vi "Share boolean signal.vi"() -> ()   [LabVIEW 2012]
uses:
  <vilib>/Platform/TimedLoop/XDataNode/timing_clust.ctl
  <vilib>/Platform/TimedLoop/XDataNode/nitl_modes.ctl
  <vilib>/Platform/TimedLoop/XDataNode/wakeup.ctl
  <vilib>/rvi/Emulation/niFpgaSctlEmulationRegisterWithScheduler.vi
  <vilib>/rvi/Emulation/niFpgaSctlEmulationScheduler.vi
  <vilib>/Platform/TimedLoop/XDataNode/XDataNode.xnode
  <vilib>/Platform/TimedLoop/XDataNode/XDNodeRunTimeDep.lvlib
panel:
  out "Falling Edge Trigger LED":bool
  out "Rising Edge Trigger LED":bool
  in  "Count (ms)":u32=2000
  in  "stop":bool
  out "Generated Clock":bool
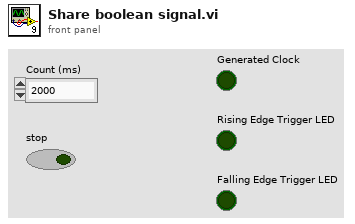
[diagram p1: front panel]
types:
  T1 = typedef "XDNodeRunTimeDep.lvlib/timing_clust.ctl" = cluster{"Expected End [f-1]":u64, "Actual End [f-1]":u64, "Finished Late? [f-1]":bool, "Expected End [i-1]":u64, "Actual End [i-1]":u64, "Finished Late? [i-1]":bool, "Expected Start [i]":u64, "Actual Start [i]":u64, "Expected Start [f]":u64, "Actual Start [f]":u64, "Source Name":string, "Structure Name":string, "Period":i64, "Deadline":i64, "Offset":i64, "Start":i64, "Priority":i32, "Timeout":i32, "Mode":T2, "Wakeup Reason":T3, "Error":errorcluster, "Source Type":string, "Secondary Source Type":string, "Global End Time":u64, "Global Start Time":u64, "Frame Duration":u64, "Iteration Duration":u64, "Assigned CPU":i32, "I/O Scan Engine Mode":u32}
  T2 = typedef "XDNodeRunTimeDep.lvlib/nitl_modes.ctl" = enum32{"No Change", "Process missed periods, maintain original phase", "Discard missed periods, maintain original phase", "Process missed periods, ignore original phase", "Discard missed periods, ignore original phase"}
  T3 = typedef "XDNodeRunTimeDep.lvlib/wakeup.ctl" = enum32{"Normal", "Aborted", "Asynchronous wakeup", "Timing source error", "Timed loop error", "Timeout"}
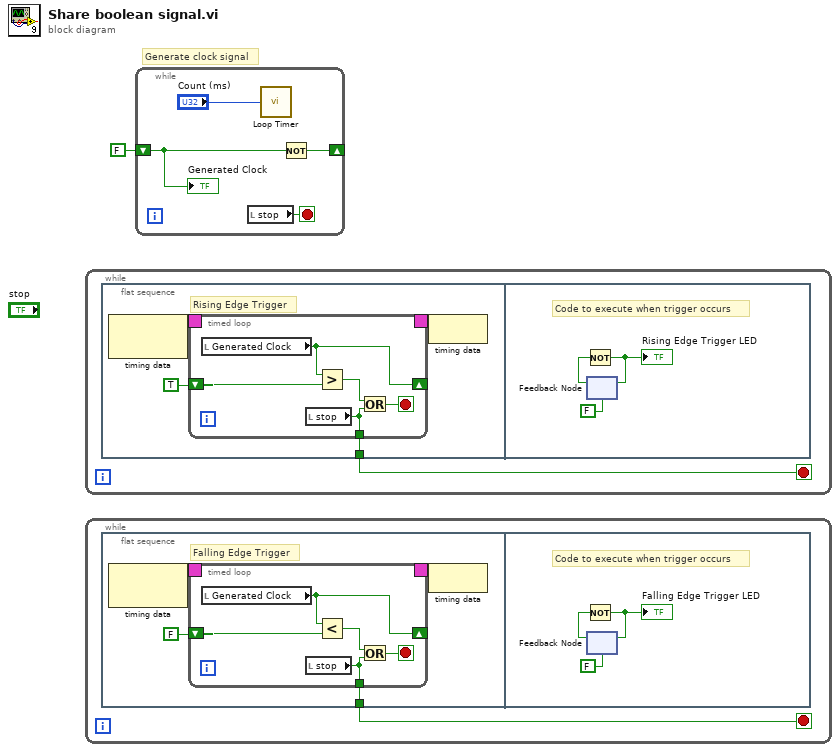
[diagram p0: block diagram]
diagram:
  # "Generate clock signal"
  n1 = while {
    stop <- w2 stop-if-true
    n2 = flat-sequence {
      tunnel: [w3] -> w2
      frame #0 {
        # "Rising Edge Trigger"
        n3 = node-c288 ("Rising Edge Trigger")() -> (w6:T1)  [unwired: 1 in]
        n4 = timed-loop "Rising Edge Trigger" {
          timing: w6 -> [_]
          timing-out: [_] -> w5
          shift-right: [w10] -> _
          shift-left: TRUE -> [w11]
          tunnel: [w7] -> w3
          stop <- w8 stop-if-true
          n5 = local read "Generated Clock"() -> (w10:bool)
          n6 = local read "stop"() -> (w7:bool)
          n7 = Greater?(x=w10, y=w11) -> (0:w9:bool)
          n8 = Or(x=w9, y=w7) -> (x .or. y?=w8:bool)
        }
        n9 = node-c288(w5) -> ()
      }
      frame #1 {
        # "Code to execute when trigger occurs"
        n10 = feedback #1(FALSE) -> (w18:bool)
        n11 = Not(x=w18) -> (.not. x?=w17:bool)
        "Rising Edge Trigger LED" <- w17
        n12 = feedback-in #1(w17) -> ()
      }
    }
  }
  n13 = while {
    stop <- w19 stop-if-true
    n14 = flat-sequence {
      tunnel: [w20] -> w19
      frame #0 {
        # "Falling Edge Trigger"
        n15 = node-c288 ("Rising Edge Trigger")() -> (w23:T1)  [unwired: 1 in]
        n16 = timed-loop "Falling Edge Trigger" {
          timing: w23 -> [_]
          timing-out: [_] -> w22
          shift-right: [w27] -> _
          shift-left: FALSE -> [w28]
          tunnel: [w24] -> w20
          stop <- w25 stop-if-true
          n17 = local read "Generated Clock"() -> (w27:bool)
          n18 = local read "stop"() -> (w24:bool)
          n19 = Less?(x=w27, y=w28) -> (x < y?=w26:bool)
          n20 = Or(x=w26, y=w24) -> (x .or. y?=w25:bool)
        }
        n21 = node-c288(w22) -> ()
      }
      frame #1 {
        # "Code to execute when trigger occurs"
        n22 = feedback #2(FALSE) -> (w33:bool)
        n23 = Not(x=w33) -> (.not. x?=w34:bool)
        "Falling Edge Trigger LED" <- w34
        n24 = feedback-in #2(w34) -> ()
      }
    }
  }
  n25 = while "Generate Clock Signal" {
    shift-right: [w38] -> _
    shift-left: FALSE -> [w36]
    stop <- w37 stop-if-true
    n26 = local read "stop"() -> (w37:bool)
    n27 = call "Loop Timer"("Count(mSec)"="Count (ms)") -> ()  [unwired: 1 out]
    n28 = Not(x=w36) -> (.not. x?=w38:bool)
    "Generated Clock" <- w36
  }
